vi "GPS经纬度解析 (子VI).vi"(9 "小数":u16, 10 "分":u16, 11 "度":u16) -> (3 "数值输出":dbl format="%#.6g")   [LabVIEW 2016, in "环境动力监测库.lvlib" / "NMEA.lvlib"]
uses:
  NMEA.lvlib
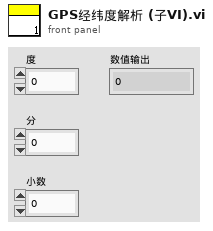
[diagram p1: front panel]
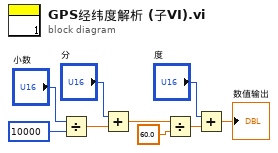
[diagram p0: block diagram]
diagram:
  n1 = Divide(x="小数", y=u16 10000) -> (x/y=w5:dbl)
  n2 = Add(x="分", y=w5) -> (x+y=w4:dbl)
  n3 = Divide(x=w4, y=60.0) -> (x/y=w2:dbl)
  n4 = Add(x="度", y=w2) -> (x+y=→"数值输出":dbl)
